vi "rateScanDone.vi"(8 "error in (no error)":errorcluster, 11 "Model in":refnum<class "Model.lvclass">) -> (0 "error out":errorcluster, 2 "Done?":bool, 3 "Model out":refnum<class "Model.lvclass">)   [LabVIEW 2015, in "Model.lvclass"]
uses:
  Model.lvclass
  Model.lvclass/Model.ctl
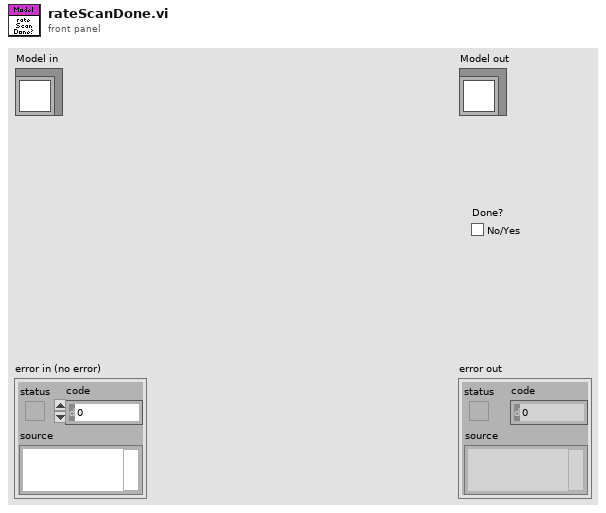
[diagram p1: front panel]
types:
  T1 = typedef "ILCCommon.lvlib/ILCConfiguration.lvlib/Scan Rates.ctl" = enum16{"50", "60", "100", "120", "200", "240", "300", "400", "480", "600", "1200", "2400", "4800"}
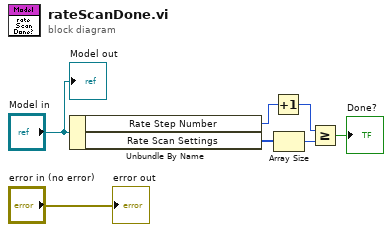
[diagram p0: block diagram]
diagram:
  n1 = Unbundle By Name("Model in") -> ("Rate Step Number"=w4:u16, "Rate Scan Settings"=w5:T1[])
  n2 = Increment(x=w4) -> (x+1=w3:u16)
  n3 = Array Size(array=w5) -> (size(s)=w2:i32)
  n4 = Greater Or Equal?(x=w3, y=w2) -> (x >= y?=→"Done?":bool)
  "error out" <- "error in (no error)"
  "Model out" <- "Model in"
